vi "20220110_MultiFuncGen.vi"() -> ()   [LabVIEW 2021]
doc: "This example demonstrates how to generate a user-defined voltage using the analog output of a DAQ device."
uses:
  <vilib>/Utility/error.llb/DialogType.ctl
  <vilib>/DAQmx/write.llb/DAQmx Write (Analog 1D DBL NChan 1Samp).vi
  <vilib>/DAQmx/write.llb/DAQmx Write (Digital U8 1Chan 1Samp).vi
  <vilib>/DAQmx/create/channels.llb/DAQmx Create Channel (AO-Voltage-Basic).vi
  <vilib>/DAQmx/create/channels.llb/DAQmx Create Channel (DO-Digital Output).vi
  <vilib>/Utility/file.llb/Read Delimited Spreadsheet (DBL).vi
  <vilib>/DAQmx/miscellaneous.llb/DAQmx Fill In Error Info.vi
panel:
  in  "value":bool
  out "AO":T1(graph)
  out "DIO":cluster{i16, i16, i16, i16, i16}(graph)
  in  "file path (dialog if empty)":path
  in  "DO":tag
  in  "AO":tag
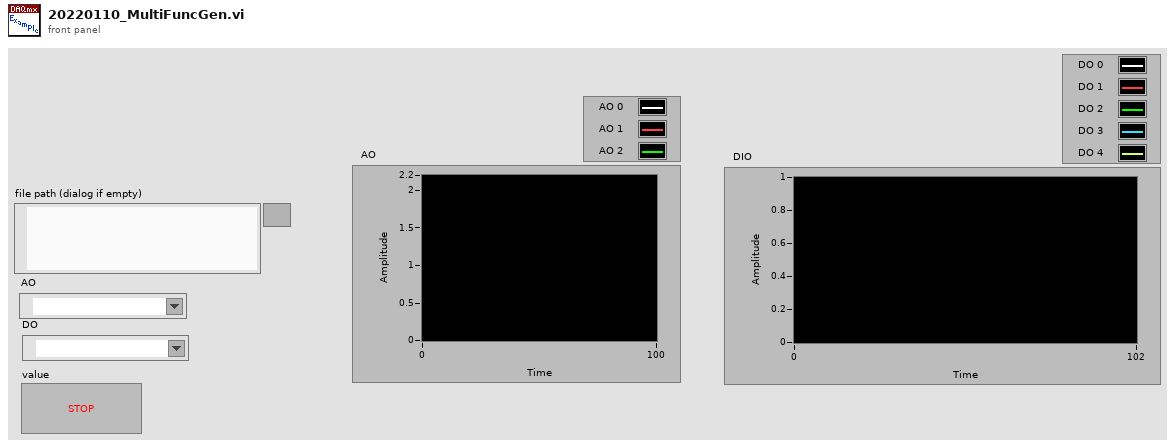
[diagram p1: front panel]
types:
  T1 = cluster{"Numeric":dbl, "Numeric":dbl, "Numeric":dbl}
  T2 = typedef "DialogType.ctl" = u16
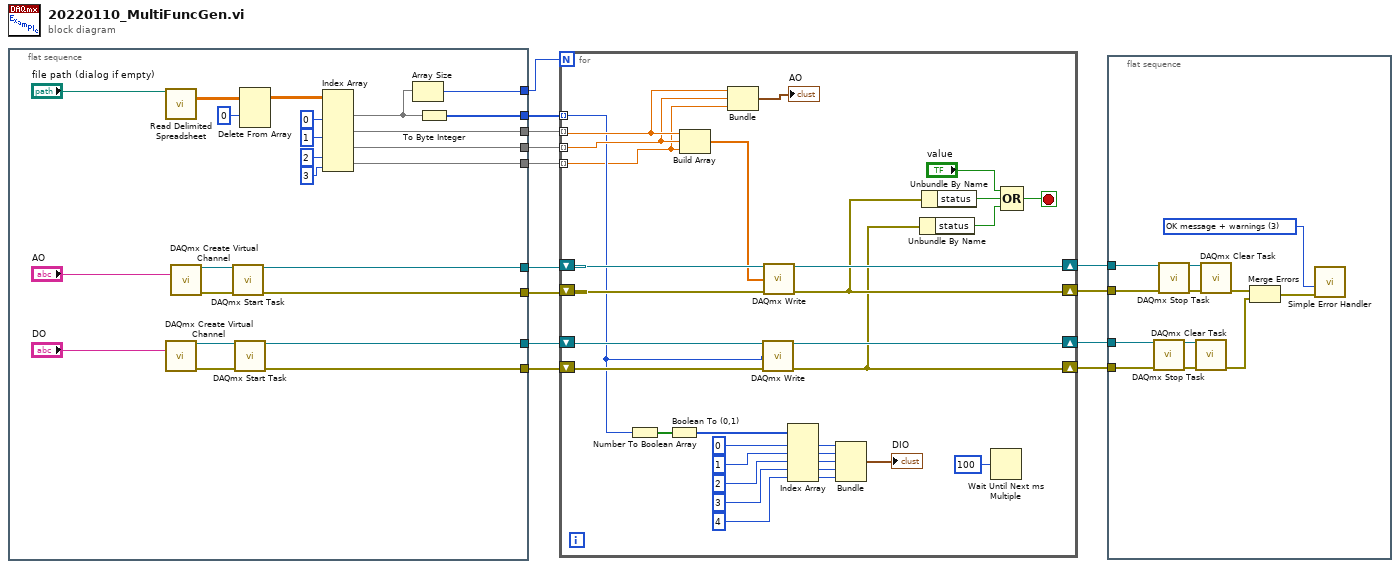
[diagram p0: block diagram]
diagram:
  n1 = flat-sequence {
    tunnel: [w35] -> w13
    tunnel: [w34] -> w12
    tunnel: [w31] -> w9
    tunnel: [w30] -> w8
    tunnel: [w19] -> w5
    tunnel: [w18] -> w4
    tunnel: [w17] -> w3
    tunnel: [w16] -> w2
    tunnel: [w14] -> w1
    frame #0 {
      n2 = call-poly <vilib>:"Read Delimited Spreadsheet.vi"("file path (dialog if empty)"="file path (dialog if empty)") -> ("all rows"=w26:dbl[][])  [unwired: 9 in, 5 out]
      n3 = call-poly <vilib>:"DAQmx Create Virtual Channel.vi"("lines"="DO") -> ("task out"=w33:refnum<k21>, "error out"=w32:errorcluster)  [unwired: 13 in]
      n4 = call-poly <vilib>:"DAQmx Create Virtual Channel.vi"("physical channels"="AO") -> ("task out"=w37:refnum<k21>, "error out"=w36:errorcluster)  [unwired: 13 in]
      n5 = call <vilib>:"DAQmx Start Task.vi"("task/channels in"=w37, "error in"=w36) -> ("task out"=w35:refnum<k21>, "error out"=w34:errorcluster)  [unwired: 12 in]
      n6 = call <vilib>:"DAQmx Start Task.vi"("task/channels in"=w33, "error in"=w32) -> ("task out"=w31:refnum<k21>, "error out"=w30:errorcluster)  [unwired: 12 in]
      n7 = Delete From Array(array=w26, index (row)=0) -> (array with subset deleted=w24:dbl[][])  [unwired: 2 in, 1 out]
      n8 = Index Array(array=w24, index (col) #1=0 ("disabled index (col)"), index (col) #2=1 ("index (col)"), index (col) #3=2 ("index (col)"), index (col) #4=3 ("index (col)")) -> (element #1=w20:dbl[], element #2=w17:dbl[], element #3=w16:dbl[], element #4=w14:dbl[])  [unwired: 4 in]
      n9 = Array Size(array=w20) -> (size(s)=w19:i32)
      n10 = To Byte Integer(number=w20) -> (8bit integer=w18:i8[])
    }
  }
  n11 = for {
    N: w5 -> [_]
    shift-right: [w67] -> w11
    shift-left: w13 -> [w69]
    shift-right: [w45] -> w10
    shift-left: w12 -> [w68]
    shift-right: [w64] -> w7
    shift-left: w9 -> [w66]
    shift-right: [w44] -> w6
    shift-left: w8 -> [w65]
    tunnel: w4 -> [w42] mode=indexing
    tunnel: w3 -> [w49] mode=indexing
    tunnel: w2 -> [w48] mode=indexing
    tunnel: w1 -> [w38] mode=indexing
    stop <- w43 stop-if-true
    n12 = Number To Boolean Array(number=w42) -> (Boolean array=w41:bool[])
    n13 = Boolean To (0,1)(Boolean=w41) -> (0, 1=w61:i16[])
    n14 = Build Array(w49, w48, w38) -> (w62:dbl[])
    n15 = Bundle("Numeric"=w49, "Numeric"=w48, "Numeric"=w38) -> (→"AO":T1)  [unwired: 1 in]
    n16 = call-poly <vilib>:"DAQmx Write.vi"("task/channels in"=w66, "data"=w42, "error in"=w65) -> ("task out"=w64:refnum<k21>, "error out"=w44:errorcluster)  [unwired: 10 in, 1 out]
    n17 = call-poly <vilib>:"DAQmx Write.vi"("task/channels in"=w69, "data"=w62, "error in"=w68) -> ("task out"=w67:refnum<k21>, "error out"=w45:errorcluster)  [unwired: 10 in, 1 out]
    n18 = Index Array(array=w61, index #1=0 ("index"), index #2=1 ("index"), index #3=2 ("index"), index #4=3 ("index"), index #5=4 ("index")) -> (element #1=w55:i16, element #2=w54:i16, element #3=w53:i16, element #4=w52:i16, element #5=w51:i16)
    n19 = Bundle(w55, w54, w53, w52, w51) -> (→"DIO":cluster{i16, i16, i16, i16, i16})  [unwired: 1 in]
    n20 = Unbundle By Name(w44) -> ("status"=w46:bool)
    n21 = Unbundle By Name(w45) -> ("status"=w40:bool)
    n22 = Wait Until Next ms Multiple(millisecond multiple=u32 100) -> ()  [unwired: 1 out]
    n23 = Compound Arithmetic op=OR("value", w40, w46) -> (w43:bool)
  }
  n24 = flat-sequence {
    tunnel: w11 -> [w81]
    tunnel: w10 -> [w80]
    tunnel: w7 -> [w74]
    tunnel: w6 -> [w73]
    frame #0 {
      w77 = T2 3 items=["no dialog", "OK message", "continue or stop message", "OK message + warnings", "continue/stop + warnings"] ("type of dialog (OK msg:1)")
      n25 = call <vilib>:"DAQmx Stop Task.vi"("task/channels in"=w74, "error in"=w73) -> ("task out"=w75:refnum<k21>, "error out"=w76:errorcluster)  [unwired: 12 in]
      n26 = call <vilib>:"DAQmx Stop Task.vi"("task/channels in"=w81, "error in"=w80) -> ("task out"=w79:refnum<k21>, "error out"=w78:errorcluster)  [unwired: 12 in]
      n27 = call <vilib>:"DAQmx Clear Task.vi"("task in"=w75, "error in"=w76) -> ("error out"=w70:errorcluster)  [unwired: 13 in]
      n28 = call <vilib>:"DAQmx Clear Task.vi"("task in"=w79, "error in"=w78) -> ("error out"=w71:errorcluster)  [unwired: 13 in]
      n29 = Merge Errors(w71, w70) -> (w72:errorcluster)
      n30 = call <vilib>:"Simple Error Handler.vi"("type of dialog (OK msg:1)"=w77, "error in (no error)"=w72) -> ()  [unwired: 3 in, 5 out]
    }
  }
